vi "Count.vi"(11 "Data In":T1) -> (3 "Data Out":T1)   [LabVIEW 2014]
uses:
  controls/Data.ctl
panel:
  # "日期"
  # "機種名稱"
  # "機種代號"
  # "商品條碼"
  # "台"
  # "OK"
  # "NG"
  # "台"
  # "總計"
  # "台"
  # "日期"
  # "機種名稱"
  # "機種代號"
  # "商品條碼"
  # "台"
  # "OK"
  # "NG"
  # "台"
  # "總計"
  # "台"
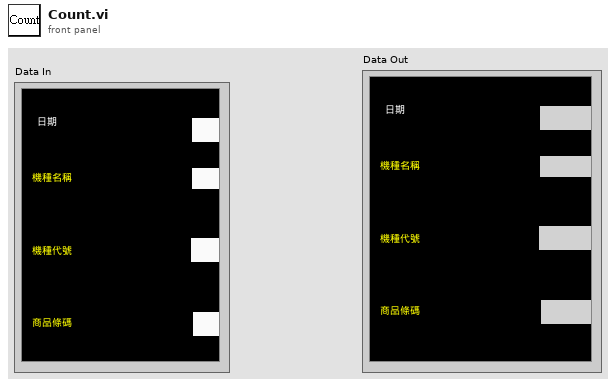
[diagram p1: front panel]
types:
  T1 = typedef "Data.ctl" = cluster{"Date":string, "BarCode1":string, "BarCode2":string, "BarCode3":string, "Message":string, "OK Count":u16, "NG Count":u16, "Total Count":u16, "ModelData":string[][], "OK&NG":bool, "COM1":refnum<visa-resource-name>, "COM2":refnum<visa-resource-name>, "IO":i32, "Time":u32, "TCP":refnum<k5>, "TCP 2":refnum<k5>}
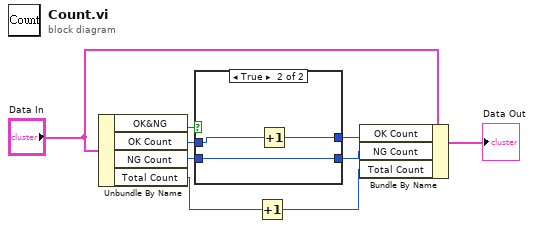
[diagram p0: block diagram]
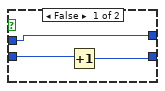
[diagram p2: hidden frame]
diagram:
  n1 = Unbundle By Name("Data In") -> ("OK&NG"=w9:bool, "OK Count"=w6:u16, "NG Count"=w4:u16, "Total Count"=w2:u16)
  n2 = case shown="True" w9 {
    tunnel: w6 -> [w12 w15]
    tunnel: [w12 w14] -> w5
    tunnel: w4 -> [w11 w13]
    tunnel: [w10 w13] -> w3
    frame False {
      n3 = Increment(x=w11) -> (x+1=w10:u16)
    }
    frame True {
      n4 = Increment(x=w15) -> (x+1=w14:u16)
    }
  }
  n5 = Increment(x=w2) -> (x+1=w1:u16)
  n6 = Bundle By Name(cluster="Data In", "OK Count"=w5, "NG Count"=w3, "Total Count"=w1) -> (→"Data Out":T1)
